vi "Motors_Encoders_Sensors_v2.vi"(0 "Speed M1 A":dbl(slide)=0.5 scale=-1.0..1.0, 1 "Speed M0 A":dbl(slide)=0.5 scale=-1.0..1.0, 2 "Reset All Encoders":bool, 5 "Speed M1 B":dbl(slide)=0.5 scale=-1.0..1.0, 7 "Speed M0 B":dbl(slide)=0.5 scale=-1.0..1.0, 9 "Invert M1 B":bool, 11 "Invert M0 B":bool, 12 "Invert M0 A":bool, 13 "Invert M1 A":bool) -> (3 "Distance M0 A(cm)":dbl, 4 "Distance M1 A(cm)":dbl, 6 "PING)))) A CM":fxp<+,64,16>, 8 "PING)))) B CM":fxp<+,64,16>, 10 "Distance M0 B(cm)":dbl, 14 "Sharp IR Distance":dbl, 15 "Distance M1 B(cm)":dbl)   [LabVIEW 2018]
uses:
  <vilib>/Studica/Studica Toolkit/Background/Mxp Selection.ctl
  <vilib>/myRIO/Common/Instrument Driver Framework/myRIO v1.0/AI/typedefs/AI Channels List.ctl
  <vilib>/myRIO/Common/Instrument Driver Framework/myRIO v1.0/AI/typedefs/AI Channels Enum.ctl
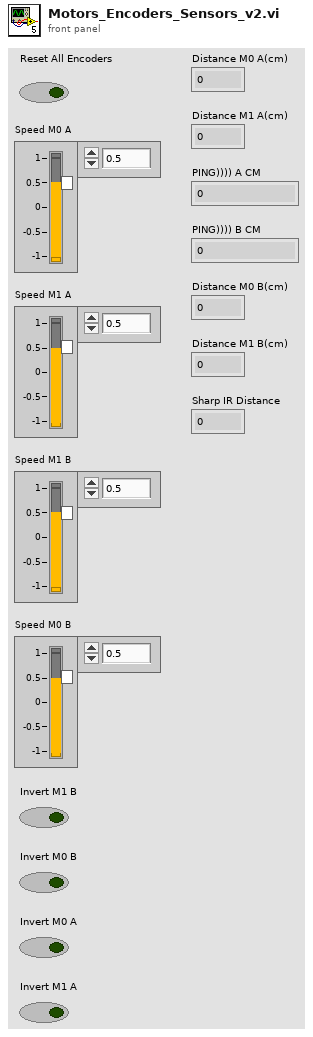
[diagram p1: front panel]
types:
  T1 = typedef "AI Channels List.ctl" = T2[]
  T2 = typedef "AI Channels Enum.ctl" = enum16{"Not Connected", "AudioIn/Left", "AudioIn/Right", "C/AI0", "C/AI1", "A/AI0", "A/AI1", "A/AI2", "A/AI3", "A/AI4", "A/AI5", "A/AI6", "A/AI7", "B/AI0", "B/AI1", "B/AI2", "B/AI3", "B/AI4", "B/AI5", "B/AI6", "B/AI7", "AI/AI0", "AI/AI1", "AI/AI2", "AI/AI3", "A/AI0 (DIFF)", "A/AI1 (DIFF)", "A/AI2 (DIFF)", "A/AI3 (DIFF)", "B/AI0 (DIFF)", "B/AI1 (DIFF)", "B/AI2 (DIFF)", "B/AI3 (DIFF)"}
  T3 = typedef "Mxp Selection.ctl" = enum16{"MXP A", "MXP B"}
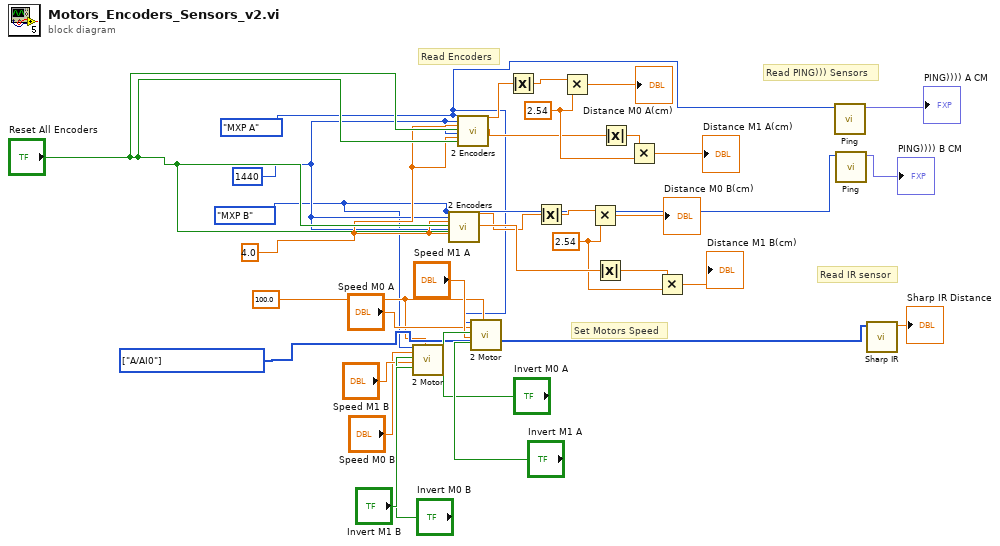
[diagram p0: block diagram]
diagram:
  w18 = 2.54 ("Frequency [Hz]")
  w13 = 2.54 ("Frequency [Hz]")
  w6 = T1 [enum."A/AI0"] items=["Not Connected", "AudioIn/Left", "AudioIn/Right", "C/AI0", "C/AI1", "A/AI0", "A/AI1", "A/AI2", "A/AI3", "A/AI4", "A/AI5", "A/AI6", "A/AI7", "B/AI0", "B/AI1", "B/AI2", "B/AI3", "B/AI4", "B/AI5", "B/AI6", "B/AI7", "AI/AI0", "AI/AI1", "AI/AI2", "AI/AI3", "A/AI0 (DIFF)", "A/AI1 (DIFF)", "A/AI2 (DIFF)", "A/AI3 (DIFF)", "B/AI0 (DIFF)", "B/AI1 (DIFF)", "B/AI2 (DIFF)", "B/AI3 (DIFF)"] ("AI Channel")
  w5 = 100.0 ("Frequency [Hz]")
  w4 = 4.0 ("Wheel Diameter M0 (inches)")
  w3 = u32 1440 ("Ticks Per Rev M0")
  w2 = Mxp_Selection."MXP B" ("Mxp Side")
  w1 = Mxp_Selection."MXP A" ("Mxp Side")
  # "Read IR sensor"
  # "Read PING))) Sensors"
  # "Set Motors Speed"
  # "Read Encoders"
  n1 = call <vilib>:"2 Motor.vi"("Mxp Side"=w2, "Speed M0"="Speed M0 B", "Invert M0"="Invert M0 B", "Speed M1"="Speed M1 B", "Invert M1"="Invert M1 B", "Frequency [Hz]"=w5) -> ()  [unwired: 13 in, 1 out]
  n2 = call <vilib>:"2 Encoders.vi"("Mxp Side"=w2, "Ticks Per Rev M0"=w3, "Wheel Diameter M0 (inches)"=w4, "Reset Encoder 0"="Reset All Encoders", "Ticks Per Rev M1"=w3, "Wheel Diameter M1 (inches)"=w4, "Reset Encoder 1"="Reset All Encoders") -> ("Distance M0 (inches)"=w19:dbl, "Distance M1 (inches)"=w20:dbl)  [unwired: 18 in, 1 out]
  n3 = call <vilib>:"2 Encoders.vi"("Mxp Side"=w1, "Ticks Per Rev M0"=w3, "Wheel Diameter M0 (inches)"=w4, "Reset Encoder 0"="Reset All Encoders", "Ticks Per Rev M1"=w3, "Wheel Diameter M1 (inches)"=w4, "Reset Encoder 1"="Reset All Encoders") -> ("Distance M0 (inches)"=w8:dbl, "Distance M1 (inches)"=w12:dbl)  [unwired: 18 in, 1 out]
  n4 = call <vilib>:"2 Motor.vi"("Mxp Side"=w1, "Speed M0"="Speed M0 A", "Invert M0"="Invert M0 A", "Speed M1"="Speed M1 A", "Invert M1"="Invert M1 A", "Frequency [Hz]"=w5) -> ()  [unwired: 13 in, 1 out]
  n5 = Absolute Value(x=w8) -> (abs(x)=w7:dbl)
  n6 = Absolute Value(x=w19) -> (abs(x)=w14:dbl)
  n7 = Multiply(x=w7, y=w13) -> (x*y=→"Distance M0 A(cm)":dbl)
  n8 = Multiply(x=w14, y=w18) -> (x*y=→"Distance M0 B(cm)":dbl)
  n9 = Absolute Value(x=w20) -> (abs(x)=w17:dbl)
  n10 = Absolute Value(x=w12) -> (abs(x)=w11:dbl)
  n11 = Multiply(x=w11, y=w13) -> (x*y=→"Distance M1 A(cm)":dbl)
  n12 = Multiply(x=w17, y=w18) -> (x*y=→"Distance M1 B(cm)":dbl)
  n13 = call <vilib>:"Ping.vi"("Mxp Side"=w1) -> ("CM"=→"PING)))) A CM":fxp<+,64,16>)  [unwired: 8 in, 2 out]
  n14 = call <vilib>:"Ping.vi"("Mxp Side"=w2) -> ("CM"=→"PING)))) B CM":fxp<+,64,16>)  [unwired: 8 in, 2 out]
  n15 = call <vilib>:"Sharp IR.vi"("AI Channel"=w6) -> ("Sharp IR Distance"=→"Sharp IR Distance":dbl)  [unwired: 8 in, 2 out]
